vi "Build Context Menu.vi"(8 "error in (no error)":errorcluster, 10 "MenuRef":refnum<k9>, 11 "HIJ IMAQdx Display in":refnum<class "HIJ IMAQdx Display.lvclass">) -> (0 "error out":errorcluster, 2 "MenuRef out":refnum<k9>, 3 "HIJ IMAQdx Display out":refnum<class "HIJ IMAQdx Display.lvclass">)   [LabVIEW 2014, in "HIJ IMAQdx Display.lvlib" / "HIJ IMAQdx Display.lvclass"]
uses:
  HIJ IMAQdx Display.lvclass
  HIJ IMAQdx Display.lvclass/HIJ IMAQdx Display.ctl
  HIJ Vision Display/HIJ Vision Display/HIJ Vision Display.lvclass
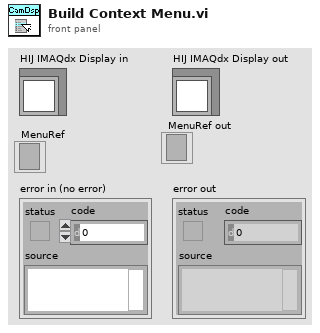
[diagram p1: front panel]
types:
  T1 = typedef "IMAQ Image.ctl" = refnum<image>
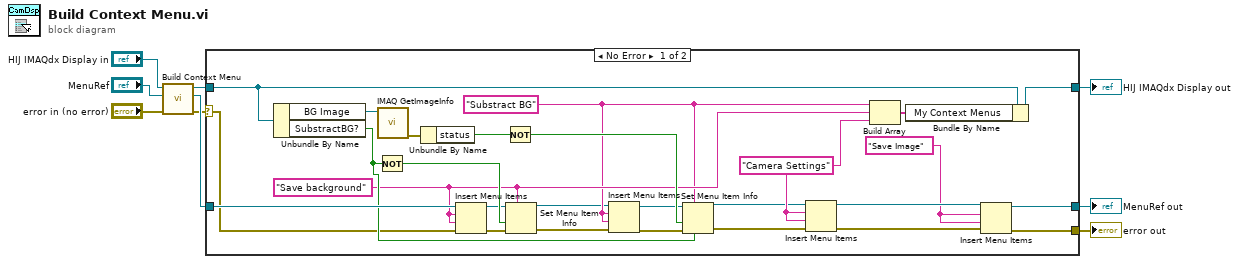
[diagram p0: block diagram]
diagram:
  n1 = call-parent "Build Context Menu.vi"("error in (no error)"="error in (no error)", "MenuRef"="MenuRef", "HIJ Vision Display in"="HIJ IMAQdx Display in") -> ("error out"=w2:errorcluster, "MenuRef out"=w5:refnum<k9>, "HIJ Vision Display out"=w6:refnum<class "HIJ IMAQdx Display.lvclass">)  [unwired: 6 in]
  n2 = case shown="No Error" w2 {
    selector: w2 -> [w24 w39]
    tunnel: w6 -> [w30 w37]
    tunnel: w5 -> [w31 w38]
    tunnel: [w11 w38] -> w4
    tunnel: [w10 w39] -> w3
    tunnel: [w29 w37] -> w1
    frame No Error {
      w12 = "Save Image" ("item tag")
      w17 = "Camera Settings" ("item tag")
      w22 = "Substract BG" ("item tag")
      w25 = "Save background" ("item tag")
      n3 = Unbundle By Name(w30) -> ("BG Image"=w32:T1, "SubstractBG?"=w27:bool)
      n4 = Not(x=w27) -> (.not. x?=w33:bool)
      n5 = call "IMAQ GetImageInfo"("Image"=w32) -> ("error out"=w35:errorcluster)  [unwired: 3 in, 7 out]
      n6 = Unbundle By Name(w35) -> ("status"=w34:bool)
      n7 = Insert Menu Items(6:w24, 7:w25, 8:w25, 9:w31) -> (0:w23:errorcluster, 3:w26:refnum<k9>)  [unwired: 2 in, 1 out]
      n8 = Not(x=w34) -> (.not. x?=w36:bool)
      n9 = Set Menu Item Info(7:w25, 8:w23, 9:w33, 11:w26) -> (0:w20:errorcluster, 3:w21:refnum<k9>)  [unwired: 3 in]
      n10 = Insert Menu Items(6:w20, 7:w22, 8:w22, 9:w21) -> (0:w18:errorcluster, 3:w19:refnum<k9>)  [unwired: 2 in, 1 out]
      n11 = Set Menu Item Info(6:w27, 7:w22, 8:w18, 9:w36, 11:w19) -> (0:w15:errorcluster, 3:w16:refnum<k9>)  [unwired: 2 in]
      n12 = Insert Menu Items(6:w15, 7:w17, 8:w17, 9:w16) -> (0:w13:errorcluster, 3:w14:refnum<k9>)  [unwired: 2 in, 1 out]
      n13 = Build Array(w22, w25, w17) -> (w28:string[])
      n14 = Bundle By Name(cluster=w30, "My Context Menus"=w28) -> (w29:refnum<class "HIJ IMAQdx Display.lvclass">)
      n15 = Insert Menu Items(6:w13, 7:w12, 8:w12, 9:w14) -> (0:w10:errorcluster, 3:w11:refnum<k9>)  [unwired: 2 in, 1 out]
    }
    frame Error {
    }
  }
  "error out" <- w3
  "HIJ IMAQdx Display out" <- w1
  "MenuRef out" <- w4
